vi "Self-Test.vi"(8 "error in (no error)":errorcluster, 11 "VISA resource name":refnum<visa-resource-name>) -> (0 "error out":errorcluster, 1 "Self-Test Result Message":string, 2 "Self-Test Result Code":i32, 3 "VISA resource name out":refnum<visa-resource-name>)   [LabVIEW 2014, in "GRBLMotionCore.lvlib"]
doc: "Runs the instrument's self-test routine and returns the test results."
uses:
  <instrlib>/GRBL/GRBLMotionCore.lvlib
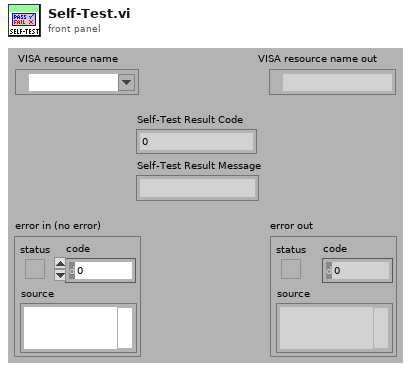
[diagram p1: front panel]
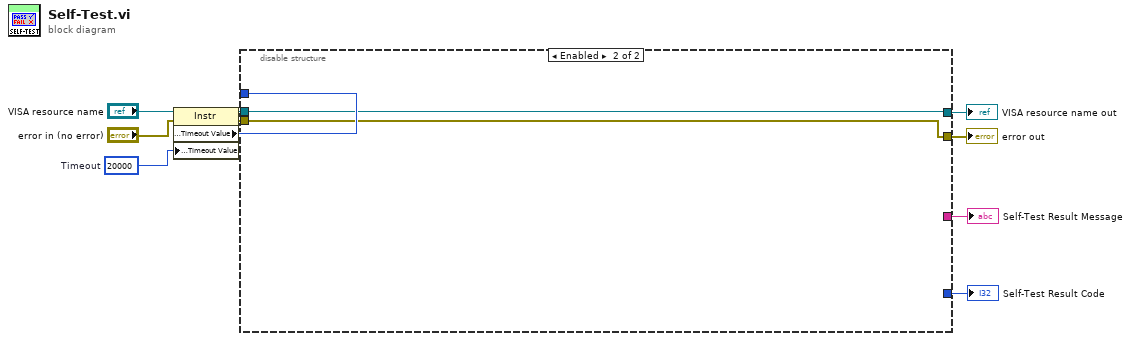
[diagram p0: block diagram]
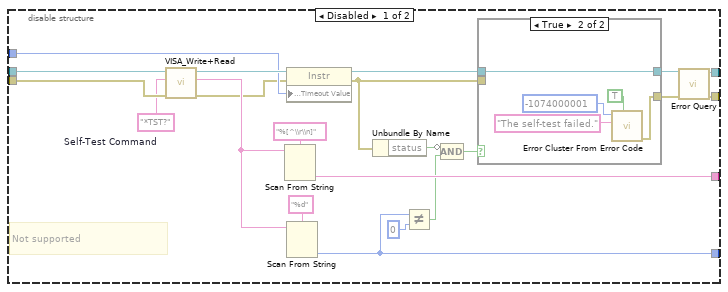
[diagram p2: hidden frame]
diagram:
  w5 = u32 20000  # Timeout
  n1 = property class="Instr"(reference="VISA resource name", error in="error in (no error)", "General Settings:Timeout Value"=w5) -> (reference out=w3:refnum<visa-resource-name>, error out=w4:errorcluster, "General Settings:Timeout Value"=w2:u32)
  n2 = disable-structure shown="Enabled" {
    disable-tunnel: [w28 w40] -> w8
    disable-tunnel: [w27 w39] -> w7
    disable-tunnel: [w26 _] -> w6
    disable-tunnel: w4 -> [w25 w39]
    disable-tunnel: w3 -> [w24 w40]
    disable-tunnel: w2 -> [w23 _]
    disable-tunnel: [w14 _] -> w1
    frame Disabled {
      w22 = "*TST?"  # Self-Test Command
      # "Not supported"
      n3 = call <instrlib>:"VISA_Write+Read.vi"("error in (no error)"=w25, "Write Buffer"=w22, "VISA resource name"=w24) -> ("error out"=w11:errorcluster, "readout"=w12:string, "VISA resource name out"=w29:refnum<visa-resource-name>)  [unwired: 6 in]
      n4 = Scan From String(format string="%[^\\r\\n]" ("Format String"), input string=w12) -> (output 1=w26:string)  [unwired: 3 in, 3 out]
      n5 = property class="Instr"(reference=w29, error in=w11, "General Settings:Timeout Value"=w23) -> (reference out=w21:refnum<visa-resource-name>, error out=w20:errorcluster)
      n6 = Scan From String(format string="%d", input string=w12) -> (output 1=w14:i32)  [unwired: 3 in, 3 out]
      n7 = Unbundle By Name(w20) -> ("status"=w16:bool)
      n8 = Not Equal?(x=w14, y=0) -> (x != y?=w17:bool)
      n9 = Compound Arithmetic op=AND(invert w16, w17) -> (w15:bool)
      n10 = case shown="True" w15 {
        tunnel: w21 -> [w33 w38]
        tunnel: w20 -> [w32 _]
        tunnel: [w32 w34] -> w19
        tunnel: [w33 w38] -> w18
        frame False {
        }
        frame True {
          n11 = call <vilib>:"Error Cluster From Error Code.vi"("show call chain? (False)"=TRUE, "error message (\"\")"="The self-test failed." ("Source (VI Name)"), "error code (0)"=-1074000001 ("Code")) -> ("error out"=w34:errorcluster)  [unwired: 6 in]
        }
      }
      n12 = call <instrlib>:"Error Query.vi"("error in (no error)"=w19, "VISA resource name"=w18) -> ("error out"=w27:errorcluster, "VISA resource name out"=w28:refnum<visa-resource-name>)  [unwired: 6 in, 2 out]
    }
    frame Enabled {
    }
  }
  "Self-Test Result Message" <- w6
  "Self-Test Result Code" <- w1
  "VISA resource name out" <- w8
  "error out" <- w7
